vi "Main.vi"() -> ()   [LabVIEW 2013] (continued)
                n3208 = property on="Chart" class="WFChart (strict)"("History Data"=dynamicdata[] [[]]) -> (error out=w5362:errorcluster)  [unwired: 2 in, 1 out]
                n3209 = for {
                  N: w5364 -> [_]
                  i -> [w5373]
                  n3210 = property on="Chart" class="WFChart (strict)"("Active Plot"=w5373, "Plot.Plot Name"="") -> ()  [unwired: 2 in, 2 out]
                }
                n3211 = disable-structure shown="Disabled" {
                  disable-tunnel: w5362 -> [w5371 _]
                  frame Disabled {
                    # "1 hour"
                    n3212 = Get Date/Time In Seconds() -> (seconds since 1Jan1904=w5370:timestamp)
                    n3213 = To Double Precision Float(number=w5370) -> (double precision float=w5369:dbl)
                    n3214 = Add(x=w5369, y=3600.0) -> (x+y=w5367:dbl)
                    n3215 = property on="Chart" class="WFChart (strict)"(error in=w5371, "XScale.Minimum"=w5369, "XScale.Maximum"=w5367, "XScale.Increment"=1.0 ("X Scale.Range:Increment"), "XScale.ScaleFit"=u8 1 ("X Scale.Scale Fit")) -> ()  [unwired: 1 in, 2 out]
                  }
                  frame Enabled {
                  }
                }
              }
            }
            n3216 = property on="Recording Duration" class="DigNum (strict)"("Value"=0.0) -> ()  [unwired: 2 in, 2 out]
            n3217 = property on="Remaining Hold Time" class="DigNum (strict)"("Value"=w5354) -> ()  [unwired: 2 in, 2 out]
            n3218 = disable-structure shown="Disabled" {
              frame Disabled {
                # "Will be updated below"
                n3219 = local write "Raw Data File"("") -> ()
              }
              frame Enabled {
              }
            }
            n3220 = property on="Recipe Stop" class="Bool"("DisabledEnum"=T30."Enabled" ("Disabled")) -> ()  [unwired: 2 in, 2 out]
            n3221 = property on="Recipe Start" class="Bool"("DisabledEnum"=T30."Disabled and Grayed Out" ("Disabled")) -> ()  [unwired: 2 in, 2 out]
            n3222 = property on="Process Completed" class="Bool (strict)"("Colors [4]"=w5348, "Value"=FALSE ("Overall Status")) -> ()  [unwired: 2 in, 2 out]
            n3223 = property on="Hold Time Completed" class="Bool (strict)"("Colors [4]"=w5345, "Value"=FALSE ("Hold Time Completed")) -> ()  [unwired: 2 in, 2 out]
            n3224 = property on="Overall Status" class="Bool (strict)"("Colors [4]"=w5348, "Value"=FALSE ("Overall Status")) -> ()  [unwired: 2 in, 2 out]
          }
        }
        n3225 = local read "Probe List"() -> (w5224:i32[])
        n3226 = Path To String(path=w5209) -> (string=w5208:string)
        n3227 = Open/Create/Replace File(file path (use dialog)=w5209, error in=w5218, operation (0:open)=T41."replace or create") -> (refnum out=w5235:refnum<file>, error out=w5233:errorcluster)  [unwired: 3 in, 1 out]
        n3228 = Array To Spreadsheet String(delimiter (Tab)=",", array=w5224, 3:"%d" ("format string")) -> (spreadsheet string=w5220:string)
        n3229 = local write "Raw Data File"(w5208) -> ()
        n3230 = Concatenate Strings("Time," ("string"), w5220) -> (w5206:string)
        n3231 = case shown="True" "DB - Transaction" {
          tunnel: w5214 -> [_ w5297]
          tunnel: w5209 -> [_ w5291]
          tunnel: w5212 -> [_ w5288]
          tunnel: w5206 -> [_ w5252]
          frame False {
          }
          frame True {
            w5299 = T62[] [enum."[StartRecordTime]", enum."[PerformedBy]", enum."[PerformedOn]", enum."[RawDataFilePath]", enum."[RawDataFileName]", enum."[OutputSetId]", enum."[SavedBy]", enum."[SavedOn]"] items=["[StartRecordTime]", "[StartRecordTemp]", "[MaxRecordedTemp]", "[MaxRecordedTempTime]", "[MinRecordedTemp]", "[MinRecordedTempTime]", "[EndRecordTemp]", "[EndRecordTime]", "[RecordedMinutes]", "[StartHoldTime]", "[StartHoldTemp]", "[HoldTimeMaxTemp]", "[HoldTimeMaxTempTime]", "[HoldTimeMinTemp]", "[HoldTimeMinTempTime]", "[EndHoldTime]", "[EndHoldTemp]", "[HoldDurationMinutes]", "[TempDiffDuringHold]", "[UnitOfTemperature]", "[PerformedBy]", "[PerformedOn]", "[IsTempWithinTol]", "[IsTimeWithinTol]", "[HoldTimePercentage]", "[ProcessStatus]", "[OverallStatus]", "[SequenceStatus]", "[Parameter1]", "[Parameter2]", "[Parameter3]", "[Parameter4]", "[Parameter5]", "[Parameter6]", "[Parameter7]", "[Parameter8]", "[Parameter9]", "[Parameter10]", "[Parameter11]", "[Parameter12]", "[Result]", "[RawDataFile]", "[RawDataFilePath]", "[RawDataFileName]", "[OutputSetId]", "[SavedBy]", "[SavedOn]", "[Inactive]"] ("v02")
            # "<A> [PlantId]\n<B> [StationId]\n<C> [TransactionNo]\n<D> [TransactionRunNo]"
            # "Using SRTRS.Execute.Item instead of SRTRS.Setup.Item"
            # "EXEC GetNewTransactionRunNo to get the latest TransactionRunNo!!"
            # "INSERT [SRTRS].[Execute].[Header], [SRTRS].[Execute].[Item] [SRTRS].[Execute.][TransactionResult], [SRTRS].[Execute.][ProcedureItem], [SRTRS].[Execute.][Active], [CMS].[Execute.][ActiveProcess]"
            n3232 = local read "DB Refnums II"() -> (w5239:T24)
            n3233 = local read "DB Refnums"() -> (w5278:T23)
            n3234 = call "DB - [Execute].[Transaction].vi"("DB.Schema.Table"="SRTRS.Execute.Header", "Transaction"=w5297, "error in (no error)"=errorcluster {"status"=FALSE, "code"=0, "source"=""}, "DB Connection"=T53 {"Open"=TRUE, "Close"=FALSE}, "Refnums"=w5278, "DB - Execute Transaction"=DB_-_Execute_Transaction_Enum."INSERT INTO [Header]" ("DB - Setup Item Enum"), "DB Refnums II"=w5239) -> ("connection reference"=w5251:T66, "Transaction"=w5284:T19, "SUMMARY"=w5283:errorcluster)  [unwired: 9 in, 1 out]
            n3235 = Unbundle By Name(w5284) -> ("TransactionRunNo"=w5273:string)
            n3236 = local write "TransactionRunNo"(w5273) -> ()
            n3237 = local write "TransactionRunNo (Execute)"(w5273) -> ()
            n3238 = global write "Global SRTRS.vi" "[TransactionRunNo]"(w5273) -> ()
            n3239 = Build Array("SRTRS.Execute.Item" ("DB.Schema.Table")) -> (w5276:string[])
            n3240 = call "DB - [Setup].[Item] (Part Details).vi"("DB - Setup Item Enum"=DB_-_Setup_Item_Enum."INSERT [Setup].[Item]", "DB.Schema.Table Array"=w5276, "Transaction"=w5284, "error in (no error)"=w5283, "DB Refnums"=w5278) -> ("Transaction"=w5281:T19, "SUMMARY"=w5282:errorcluster)  [unwired: 5 in, 4 out]
            n3241 = Strip Path(path=w5291) -> (stripped path=w5290:path, name=w5287:string)
            n3242 = Path To String(path=w5290) -> (string=w5264:string)
            n3243 = call "DB - [Execute].[Transaction].vi"("connection reference"=w5251, "DB.Schema.Table"="SRTRS.Execute.TransactionResult", "Transaction"=w5281, "error in (no error)"=w5282, "DB Connection"=T53 {"Open"=FALSE, "Close"=FALSE}, "Refnums"=w5278, "DB - Execute Transaction"=DB_-_Execute_Transaction_Enum."INSERT INTO [TransactionResult]" ("DB - Setup Item Enum"), "DB Refnums II"=w5239) -> ("connection reference"=w5250:T66, "Transaction"=w5286:T19, "SUMMARY"=w5293:errorcluster)  [unwired: 8 in, 1 out]
            n3244 = Concatenate Strings(w5264, "\\" ("string")) -> (w5262:string)
            n3245 = call "DB - [Execute].[Transaction].vi"("connection reference"=w5250, "DB.Schema.Table"="SRTRS.Execute.ProcedureItem", "Transaction"=w5286, "error in (no error)"=w5293, "DB Connection"=T53 {"Open"=FALSE, "Close"=FALSE}, "Refnums"=w5278, "DB - Execute Transaction"=DB_-_Execute_Transaction_Enum."INSERT INTO [ProcedureItem]" ("DB - Setup Item Enum"), "DB Refnums II"=w5239) -> ("connection reference"=w5249:T66, "Transaction"=w5285:T19, "SUMMARY"=w5292:errorcluster)  [unwired: 8 in, 1 out]
            n3246 = global read "Global SRTRS.vi" "Date Time Format"() -> (w5289:string)
            n3247 = global read "Global SRTRS.vi" "Logon"() -> (w5269:T21)
            n3248 = Unbundle By Name(w5269) -> ("UserID"=w5275:string)
            n3249 = Format Date/Time String(time format string (%c)=w5289, seconds (now)=w5288) -> (date/time string=w5256:string)  [unwired: 1 in]
            "[StartRecordTime]" <- w5256
            n3250 = property on="Output Set" class="CmbBox (strict)"() -> ("Value"=w5242:T5)  [unwired: 2 in, 2 out]
            n3251 = Build Array(w5256, w5275, w5256, w5262, w5287, w5242, w5275, w5256) -> (w5298:T5[])
            n3252 = call "DB - [Execute].[Transaction].vi"("connection reference"=w5249, "DB.Schema.Table"="SRTRS.Execute.TransactionResult", "Transaction"=w5285, "error in (no error)"=w5292, "DB Connection"=T53 {"Open"=FALSE, "Close"=FALSE}, "DB - Execute Transaction"=DB_-_Execute_Transaction_Enum."UPDATE [TransactionResult]" ("DB - Setup Item Enum"), "[TransactionResult] v02"=w5299, "<Values>"=w5298) -> ("connection reference"=w5248:T66, "Transaction"=w5266:T19, "SUMMARY"=w5272:errorcluster)  [unwired: 8 in, 1 out]
            n3253 = Unbundle By Name(w5266) -> ("TransactionNo"=w5258:string, "TransactionRunNo"=w5257:string)
            n3254 = Unbundle By Name(w5269) -> ("PlantID"=w5268:string, "StationID"=w5267:string)
            n3255 = local read "Enable Central Monitoring"() -> (w5261:bool)
            n3256 = Build Array(w5268, w5267, w5258, w5257) -> (w5265:string[])
            n3257 = call "DB - [Execute].[Transaction].vi"("connection reference"=w5248, "DB.Schema.Table"="SRTRS.Execute.Active", "error in (no error)"=w5272, "DB Connection"=T53 {"Open"=FALSE, "Close"=TRUE}, "DB - Execute Transaction"=DB_-_Execute_Transaction_Enum."INSERT/UPDATE [Execute].[Active]", "<Values>"=w5265) -> ("SUMMARY"=w5253:errorcluster)  [unwired: 10 in, 3 out]
            n3258 = And(x=w5261, y="DB - Active Process") -> (x .and. y?=w5260:bool)
            n3259 = case shown="True" w5260 {
              tunnel: [_ w5318] -> w5255
              tunnel: w5258 -> [_ w5331]
              tunnel: w5257 -> [_ w5330]
              tunnel: w5256 -> [_ w5310]
              tunnel: w5253 -> [_ _]
              tunnel: w5252 -> [_ w5315]
              frame False {
              }
              frame True {
                w5316 = "0"  # Start at Beginning
                w5332 = T63[] [enum."[IsActive]", enum."[TransactionNo]", enum."[TransactionRunNo]", enum."[StartRecordTime]", enum."[HoldProgressColor]", enum."[ProcessColor]", enum."[OverallColor]"] items=["[IsActive]", "[TransactionNo]", "[TransactionRunNo]", "[SequenceStatus]", "[StartRecordTime]", "[EndRecordTime]", "[StartHoldTime]", "[EndHoldTime]", "[Message1]", "[Message2]", "[HoldTimeRemaining]", "[HoldTimePercentage]", "[HoldProgressColor]", "[OrderNumbers]", "[CurrentTemp]", "[UnitOfTemperature]", "[IsAppClientLive]", "[RawDataFile]", "[RecordedMinutes]", "[FurnaceControlStatus]", "[FurnaceControlColor]", "[ControllerStatus]", "[ControllerColor]", "[IsControllerOnline]", "[ProcessColor]", "[OverallColor]", "[LastUpdatedOn]", "[LastUpdatedCmsTime]", "[Inactive]"] ("[Execute].[ActiveProcess]\n2014-10-14 14:58")
                n3260 = global read "Global SRTRS.vi" "Logon"() -> (w5336:T21)
                n3261 = Unbundle By Name(w5336) -> ("PlantID"=w5328:string, "SystemID"=w5327:string)
                n3262 = control-ref of="Hold Time Completed"() -> (w5309:refnum<vi>)
                n3263 = control-ref of="Overall Status"() -> (w5312:refnum<vi>)
                n3264 = control-ref of="Process Completed"() -> (w5313:refnum<vi>)
                n3265 = Bundle("PlantID"=w5328, "SystemID"=w5327) -> (w5317:cluster{"PlantID":string, "SystemID":string})  [unwired: 1 in]
                n3266 = call "DB - [CMS].[Execute].[ActiveProcess].vi"("Application"="SRTRS", "[PlantId],[SystemId]"=w5317, "DB Connection"=T53 {"Open"=TRUE, "Close"=FALSE}, "DB - CMS Execute ActiveProcess"=DB_-_CMS_Execute_Active_Process."INSERT INTO [Execute].[ActiveProcess]") -> ("connection reference"=w5326:T66, "SUMMARY"=w5335:errorcluster)  [unwired: 12 in, 2 out]
                n3267 = call "String - Boolean Ref Color.vi"("Bool Refnum"=w5313) -> ("Color (U32 String)"=w5314:string)  [unwired: 4 in]
                n3268 = call "String - Boolean Ref Color.vi"("Bool Refnum"=w5312) -> ("Color (U32 String)"=w5311:string)  [unwired: 4 in]
                n3269 = call "String - Boolean Ref Color.vi"("Bool Refnum"=w5309) -> ("Color (U32 String)"=w5308:string)  [unwired: 4 in]
                n3270 = Build Array("1" ("element"), w5331, w5330, w5310, w5308, w5314, w5311) -> (w5329:string[])
                n3271 = call "DB - [CMS].[Execute].[ActiveProcess].vi"("connection reference"=w5326, "Application"="SRTRS", "[PlantId],[SystemId]"=w5317, "error in (no error)"=w5335, "DB Connection"=T53 {"Open"=FALSE, "Close"=FALSE}, "DB - CMS Execute ActiveProcess"=DB_-_CMS_Execute_Active_Process."UPDATE [Execute].[ActiveProcess]", "[Execute].[ActiveProcess]\n2014-10-14 14:58"=w5332, "<Data>"=w5329) -> ("connection reference"=w5320:T66, "SUMMARY"=w5319:errorcluster)  [unwired: 8 in, 2 out]
                n3272 = call "DB - [CMS].[Execute].[ActiveProcess].vi"("connection reference"=w5320, "Application"="SRTRS", "String ([RawDataFile] Filestream)"=w5315, "[PlantId],[SystemId]"=w5317, "error in (no error)"=w5319, "DB Connection"=T53 {"Open"=FALSE, "Close"=TRUE}, "Filestream Position (0/<int>/NULL)"=w5316, "DB - CMS Execute ActiveProcess"=DB_-_CMS_Execute_Active_Process."UPDATE FILESTREAM") -> ("SUMMARY"=w5318:errorcluster)  [unwired: 8 in, 3 out]
              }
            }
            n3273 = Merge Errors(w5255, w5253) -> (w5254:errorcluster)
            n3274 = case shown="Error" w5254 {
              tunnel: " /* [SRTRS].[Execute].[Item,TransactionResult,ProcedureItem,TransactionResult], [CMS].[Execute].[ActiveProcess]*/" ("Message") -> [w5338 w5341]
              tunnel: [w5337 w5340] -> w5241
              frame No Error {
                n3275 = Concatenate Strings("{Start Recipe} Transaction DB Record Create OK." ("string"), w5338) -> (w5337:string)
              }
              frame Error {
                n3276 = Concatenate Strings("{Start Recipe} Transaction DB Record Create Failed." ("string"), w5341) -> (w5340:string)
              }
            }
            n3277 = call "Queue - EnQueue to MessageQ.vi"("<NoD> Don't Display to UI"=TRUE, "Message"=w5241) -> ()  [unwired: 9 in, 1 out]
            n3278 = local write "DB"(w5254) -> ()
          }
        }
        n3279 = Write to Text File(file (use dialog)=w5235, text=w5206, error in=w5233) -> (refnum out=→"Logged File Ref":refnum<file>, error out=w5228:errorcluster)  [unwired: 1 in, 1 out]
        "Data File Error" <- w5228
        n3280 = case shown="No Error" w5228 {
          tunnel: w5207 -> [w5386 _]
          tunnel: [w5382 "{Start Recipe} Raw Data File Create Failed." ("string")] -> w5205
          frame No Error {
            w5385 = "\""
            # "Display on Front Panel"
            n3281 = local write "Raw Data File"(w5386) -> ()
            n3282 = Concatenate Strings(w5385, w5386, w5385) -> (w5378:string)
            n3283 = call <vilib>:"Application Directory.vi"() -> ("Application Directory"=w5390:path)
            n3284 = Build Path(base path=w5390, name or relative path="SRTRS.ini" ("ini Name")) -> (appended path=w5391:path)
            n3285 = call <vilib>:"Open Config Data.vi"("create file if necessary (T)"=FALSE, "configuration file path"=w5391) -> ("error out"=w5388:errorcluster, "refnum"=w5389:T59)  [unwired: 7 in, 1 out]
            n3286 = call-poly <vilib>:"Write Key.vi"("write raw string? (F)"=TRUE, "section"="Settings", "error in (no error)"=w5388, "value"=w5386, "key"="Raw Data File", "refnum"=w5389) -> ("error out"=w5394:errorcluster, "found?"=w5395:bool, "refnum out"=w5396:T59)  [unwired: 3 in]
            n3287 = call "Msgbox - Message Handler.vi"("Short Description (When DB Not Available)"="Process Started", "Description (When DB Not Available)"="Process started successfully. Raw data is logging to " ("Short Description (When DB Not Available)"), "Post-Description"=w5378, "<.?....> Message Code"="<I 303>") -> ("MHandler Error"=w5377:errorcluster)  [unwired: 5 in, 2 out]
            n3288 = local write "MHandler"(w5377) -> ()
            n3289 = call <vilib>:"Close Config Data.vi"("error in (no error)"=w5394, "write file if changed (T)"=w5395, "refnum"=w5396) -> ("error out"=w5384:errorcluster)  [unwired: 7 in, 1 out]
            n3290 = local write "ini File Error"(w5384) -> ()
            n3291 = Concatenate Strings("{Start Recipe} Raw Data File Created: " ("string"), w5378) -> (w5382:string)
          }
          frame Error {
          }
        }
        n3292 = call "Queue - EnQueue to MessageQ.vi"("<NoD> Don't Display to UI"=TRUE, "Message"=w5205) -> ()  [unwired: 9 in, 1 out]
      }
      frame "START Recovery" {
        w5426 = T62[] [enum."[RawDataFilePath]", enum."[RawDataFileName]", enum."[StartHoldTime]", enum."[EndHoldTime]", enum."[HoldTimePercentage]", enum."[StartHoldTemp]", enum."[EndHoldTemp]"] items=["[StartRecordTime]", "[StartRecordTemp]", "[MaxRecordedTemp]", "[MaxRecordedTempTime]", "[MinRecordedTemp]", "[MinRecordedTempTime]", "[EndRecordTemp]", "[EndRecordTime]", "[RecordedMinutes]", "[StartHoldTime]", "[StartHoldTemp]", "[HoldTimeMaxTemp]", "[HoldTimeMaxTempTime]", "[HoldTimeMinTemp]", "[HoldTimeMinTempTime]", "[EndHoldTime]", "[EndHoldTemp]", "[HoldDurationMinutes]", "[TempDiffDuringHold]", "[UnitOfTemperature]", "[PerformedBy]", "[PerformedOn]", "[IsTempWithinTol]", "[IsTimeWithinTol]", "[HoldTimePercentage]", "[ProcessStatus]", "[OverallStatus]", "[SequenceStatus]", "[Parameter1]", "[Parameter2]", "[Parameter3]", "[Parameter4]", "[Parameter5]", "[Parameter6]", "[Parameter7]", "[Parameter8]", "[Parameter9]", "[Parameter10]", "[Parameter11]", "[Parameter12]", "[Result]", "[RawDataFile]", "[RawDataFilePath]", "[RawDataFileName]", "[OutputSetId]", "[SavedBy]", "[SavedOn]", "[Inactive]"] ("[TransactionResult] v02")
        w5427 = T35 [enum."Page Disabled & Grayed", enum."Page Enabled", enum."Page Disabled & Grayed", enum."Page Disabled & Grayed", enum."Page Enabled"] items=["Page Enabled", "Page Disabled", "Page Disabled & Grayed"]
        # "Recovery"
        n3293 = property on="Tab Body" class="TabCtl (strict)"() -> ("Pages"=w5428:refnum<vi>[])  [unwired: 2 in, 2 out]
        n3294 = for {
          tunnel: w5428 -> [w5564] mode=indexing
          tunnel: w5427 -> [w5563] mode=indexing
          n3295 = property class="Page"(reference=w5564, "PageEnb"=w5563) -> ()  [unwired: 1 in, 2 out]
        }
        n3296 = local read "Data Path Name (cRIO SV)"() -> (w5414:string)
        n3297 = local read "Simulate cRIO"() -> (w5416:bool)
        n3298 = local read "Data_Host"() -> (w5417:path)
        n3299 = global read "Global SRTRS.vi" "[TransactionRunNo]"() -> (w5419:string)
        n3300 = global read "Global SRTRS.vi" "[TransactionNo]"() -> (w5420:string)
        n3301 = Bundle("[TransactionNo]"=w5420, "[TransactionRunNo]"=w5419) -> (w5421:T60)  [unwired: 1 in]
        n3302 = call "DB - [Execute].[Transaction].vi"("DB.Schema.Table"="SRTRS.Execute.TransactionResult", "Transaction"=w5421, "DB - Execute Transaction"=DB_-_Execute_Transaction_Enum."SELECT [TransactionResult]", "[TransactionResult] v02"=w5426) -> ("1D Results"=w5424:string[], "SUMMARY"=w5405:errorcluster)  [unwired: 12 in, 2 out]
        n3303 = local write "DB"(w5405) -> ()
        n3304 = Index Array(array=w5424) -> (element #1=w5423:string, element #2=w5422:string, element #3=w5409:string, element #4=w5408:string, element #5=w5412:string, element #6=w5407:string, element #7=w5406:string)  [unwired: 7 in]
        n3305 = Concatenate Strings(w5423, w5422) -> (w5413:string)
        n3306 = local write "Raw Data File"(w5413) -> ()
        n3307 = case shown="True" w5416 {
          tunnel: w5413 -> [w5485 w5519]
          tunnel: [w5500 w5527] -> w5415
          tunnel: [w5497 errorcluster {"status"=FALSE, "code"=0, "source"="FTP Skipped"} ("error out")] -> w5400
          tunnel: w5417 -> [w5498 _]
          tunnel: w5414 -> [w5494 _]
          frame False {
            w5479 = "\"" ("string")
            w5483 = "\"" ("string")
            # "Should Match with Raw Data File Stored in ini\nMatching ONLY the name"
            # "Change \n/c/ni-rt/LabVIEW Data/SRTRS4070/Data/2014/08/0090300742_20140822_114859.dat\nTO\nc:\\ni-rt\\LabVIEW Data\\SRTRS4070\\Data\\2014\\04\\0090300742_20140822_114859.dat"
            # "FTP Raw Data File  from cRIO AND \nReplaces data file in Data_Host\nSimilar Step as {END Recipe}"
            n3308 = Search and Replace String(replace all?=TRUE ("replace all? (F)"), input string=w5494, search string="/", replace string="\\" ("replace string (\"\")")) -> (result string=w5503:string)  [unwired: 4 in, 3 out]
            n3309 = String To Path(string=w5485) -> (path=w5487:path)
            n3310 = Strip Path "<>.dat"(path=w5487) -> (name=w5486:string)  [unwired: 1 out]
            n3311 = Search and Replace String(input string=w5503, search string="\\c", replace string="c:" ("replace string (\"\")")) -> (result string=w5478:string)  [unwired: 5 in, 3 out]
            n3312 = String To Path(string=w5478) -> (path=w5499:path)
            n3313 = Strip Path "<>.dat"(path=w5499) -> (name=w5493:string)  [unwired: 1 out]
            n3314 = Equal?(x=w5493, y=w5486) -> (x = y?=w5492:bool)
            "SV and ini Data File Name Match. (Recovery)" <- w5492
            n3315 = Build Path(base path=w5498, name or relative path=w5493) -> (appended path=w5500:path)
            n3316 = Concatenate Strings(w5479, w5478, w5479) -> (w5477:string)
            n3317 = local read "cRIO IP"() -> (w5507:string)
            n3318 = call <vilib>:"FTP Get File.vi"("password"="", "user"="anonymous", "local path"=w5500, "remote path"=w5478, "host"=w5507) -> ("error out"=w5497:errorcluster)  [unwired: 5 in, 1 out]
            n3319 = case shown="No Error" w5497 {
              tunnel: ["{Start Recovery} FTP OK. " "{Start Recovery} FTP failed. "] -> w5495
              tunnel: ["<I 321>" ("<.?....> Message Code") "<E 322>" ("<.?....> Message Code")] -> w5480
              tunnel: ["Raw Data Loaded Successfully" ("<.?....> Message Code") "Raw Data Load Failed" ("<.?....> Message Code")] -> w5476
              tunnel: [" is loaded." ("<.?....> Message Code") " cannot be loaded." ("<.?....> Message Code")] -> w5475
              frame No Error {
              }
              frame Error {
              }
            }
            n3320 = Select(t=". SV and ini Data File Name Match. ", s=w5492, f=". SV and ini Data File Name does not Match. ") -> (s? t:f=w5488:string)
            n3321 = call "Msgbox - Message Handler.vi"("Short Description (When DB Not Available)"=w5476, "Description (When DB Not Available)"=w5475, "Pre-Description"=w5477, "<.?....> Message Code"=w5480) -> ("MHandler Error"=w5481:errorcluster)  [unwired: 5 in, 2 out]
            n3322 = Concatenate Strings(w5495, "cRIO File: " ("string"), w5477, " ini File: " ("string"), w5483, w5485, w5483, w5488) -> (w5482:string)
            n3323 = local write "MHandler"(w5481) -> ()
            n3324 = call "Queue - EnQueue to MessageQ.vi"("<NoD> Don't Display to UI"=TRUE, "Message"=w5482) -> ()  [unwired: 9 in, 1 out]
          }
          frame True {
            w5521 = "\"" ("string")
            # "c:\\temp\\SRTRS4070_Host\\Data_Host\\2014\\08\\0090300742_20140822_114859.dat"
            # "Skip FTP in Simulate cRIO Mode\nRaw Data file is using the original data file in Data_Host"
            n3325 = String To Path(string=w5519) -> (path=w5527:path)
            n3326 = Concatenate Strings(w5521, w5519, w5521, " (Simulated)" ("string")) -> (w5520:string)
            n3327 = call "Msgbox - Message Handler.vi"("Short Description (When DB Not Available)"="Raw Data Loaded Successfully" ("<.?....> Message Code"), "Description (When DB Not Available)"=" is loaded." ("<.?....> Message Code"), "Pre-Description"=w5520, "<.?....> Message Code"="<I 321>") -> ("MHandler Error"=w5525:errorcluster)  [unwired: 5 in, 2 out]
            n3328 = call "Queue - EnQueue to MessageQ.vi"("<NoD> Don't Display to UI"=TRUE, "Message"="{Start Recovery} FTP skipped in cRIO Simulate Mode. ") -> ()  [unwired: 9 in, 1 out]
            n3329 = local write "MHandler"(w5525) -> ()
          }
        }
        n3330 = local read "DB - Active Process"() -> (w5403:bool)
        n3331 = local read "Enable Central Monitoring"() -> (w5404:bool)
        n3332 = flat-sequence "EXECUTE TAB" {
          tunnel: w5409 -> [w5542]
          tunnel: w5408 -> [w5541]
          tunnel: w5412 -> [w5538]
          frame #0 {
            w5544 = T36 [{"Color Box"=9868950, "Color Box 2"=9868950}, {"Color Box"=6618880, "Color Box 2"=6618880}, {"Color Box"=4934475, "Color Box 2"=4934475}, {"Color Box"=6618880, "Color Box 2"=6618880}]  # Init
            w5545 = T36 [{"Color Box"=9868950, "Color Box 2"=9868950}, {"Color Box"=6618880, "Color Box 2"=6618880}, {"Color Box"=4934475, "Color Box 2"=4934475}, {"Color Box"=6618880, "Color Box 2"=6618880}]  # Init
            w5547 = cluster{"Color Box":u32, "Color Box 2":u32}[] [{"Color Box"=16383786, "Color Box 2"=16383786}, {"Color Box"=6618880, "Color Box 2"=6618880}, {"Color Box"=4934475, "Color Box 2"=4934475}, {"Color Box"=6618880, "Color Box 2"=6618880}]  # Start Recipe
            # "Jump to Execute TAB\nThis is used when SRTRS is\nrecovered"
            # "\"START Recovery\""
            n3333 = Fract/Exp String To Number(string=w5538) -> (number=w5530:dbl)  [unwired: 3 in, 1 out]
            n3334 = call "String - Convert Str (YYYY-mm-dd HHcMMcSS) to TimeStamp.vi"("YYYY-mm-dd HH:MM:SS (String)"=w5542) -> ("time stamp"=w5540:timestamp)  [unwired: 9 in, 1 out]
            n3335 = call "String - Convert Str (YYYY-mm-dd HHcMMcSS) to TimeStamp.vi"("YYYY-mm-dd HH:MM:SS (String)"=w5541) -> ("time stamp"=w5539:timestamp)  [unwired: 9 in, 1 out]
            n3336 = Greater Or Equal?(x=w5530, y=99.5) -> (x >= y?=w5536:bool)
            n3337 = Greater?(x=w5530, y=0.0) -> (0:w5534:bool)
            n3338 = property on="Variant Allowed (Hold Temp)" class="Bool (strict)"("Colors [4]"=w5545, "Value"=FALSE) -> ()  [unwired: 2 in, 2 out]
            n3339 = local write "% Hold. Time Completed (Num)"(w5530) -> ()
            n3340 = local write "Parameter (Start Dwell Time)"(w5540) -> ()
            n3341 = local write "Parameter (End Dwell Time)"(w5539) -> ()
            n3342 = property on="Variant Allowed (Hold Time)" class="Bool (strict)"("Colors [4]"=w5545, "Value"=FALSE) -> ()  [unwired: 2 in, 2 out]
            n3343 = Select(t=u32 786176 ("Fill Color"), s=w5534, f=u32 16777216 ("Color Box 2")) -> (s? t:f=w5531:u32)
            n3344 = property on="% Hold. Time Completed" class="Slide (strict)"("Scale.Maximum"=100.0 ("Scale.Range:Maximum"), "Scale.Minimum"=0.0 ("Scale.Range:Minimum"), "Fill Color"=w5531, "Value"=w5530) -> ()  [unwired: 2 in, 2 out]
            n3345 = property on="Hold. Time (hour:minute)" class="Str"() -> ("Value"=w5555:string)  [unwired: 2 in, 2 out]
            n3346 = property on="Tab Body" class="TabCtl (strict)"("Value"=Enum_-_Tabs."Execute" ("Tab Body")) -> ()  [unwired: 2 in, 2 out]
            n3347 = call "String - Format to (HH_colon_MM).vi"("xx:xx"=w5555) -> ("seconds"=w5553:dbl)  [unwired: 9 in, 1 out]
            n3348 = flat-sequence {
              frame #0 {
                w5559 = 12  # 12 Probes Max
                n3349 = property on="Chart" class="WFChart (strict)"("History Data"=dynamicdata[] []) -> ()  [unwired: 2 in, 2 out]
                n3350 = for {
                  N: w5559 -> [_]
                  i -> [w5561]
                  n3351 = property on="Chart" class="WFChart (strict)"("Active Plot"=w5561, "Plot.Plot Name"="") -> ()  [unwired: 2 in, 2 out]
                }
              }
            }
            n3352 = property on="Recording Duration" class="DigNum (strict)"("Value"=0.0) -> ()  [unwired: 2 in, 2 out]
            n3353 = property on="Remaining Hold Time" class="DigNum (strict)"("Value"=w5553) -> ()  [unwired: 2 in, 2 out]
            n3354 = disable-structure shown="Disabled" {
              frame Disabled {
                # "Will be updated below"
                n3355 = local write "Raw Data File"("") -> ()
              }
              frame Enabled {
              }
            }
            n3356 = property on="Recipe Stop" class="Bool"("DisabledEnum"=T30."Enabled" ("Disabled")) -> ()  [unwired: 2 in, 2 out]
            n3357 = property on="Recipe Start" class="Bool"("DisabledEnum"=T30."Disabled and Grayed Out" ("Disabled")) -> ()  [unwired: 2 in, 2 out]
            n3358 = property on="Hold Time Completed" class="Bool (strict)"("Colors [4]"=w5544, "Value"=w5536) -> ()  [unwired: 2 in, 2 out]
            n3359 = property on="Process Completed" class="Bool (strict)"("Colors [4]"=w5547, "Value"=FALSE ("Overall Status")) -> ()  [unwired: 2 in, 2 out]
            n3360 = property on="Overall Status" class="Bool (strict)"("Colors [4]"=w5547, "Value"=FALSE ("Overall Status")) -> ()  [unwired: 2 in, 2 out]
          }
        }
        n3361 = Bundle By Name(cluster=T15 {"Start Holding Time and Date"="", "End Holding Time and Date"="", "Start Holding Temperature"="", "End Holding Temperature"=""} ("Parameter Buffer"), "Start Holding Time and Date"=w5409, "End Holding Time and Date"=w5408, "Start Holding Temperature"=w5407, "End Holding Temperature"=w5406) -> (w5410:T15)
        n3362 = And(x=w5404, y=w5403) -> (x .and. y?=w5402:bool)
        n3363 = property on="Parameter Buffer" class="Clust (strict)"("Value"=w5410) -> ()  [unwired: 2 in, 2 out]
        n3364 = case shown="No Error" w5400 {
          selector: w5400 -> [_ w5474]
          tunnel: w5415 -> [w5462 _]
          tunnel: [w5459 w5474] -> _
          tunnel: [w5454 refnum<file> refnum ("refnum")] -> w5401
          frame No Error {
            w5460 = "\n"
            w5449 = "\"" ("string")
            # "Shift Pointer to End of File"
            # "Overwrite raw data from cRIO to Chart"
            n3365 = call "Chart - Load History.vi"("file path (dialog if empty)"=w5462) -> ("Error Out"=w5465:errorcluster, "History"=w5466:dynamicdata[], "size(s)"=→"Recovered Data Size":i32[])  [unwired: 5 in, 3 out]
            n3366 = Path To String(path=w5462) -> (string=w5450:string)
            n3367 = property on="Chart" class="WFChart (strict)"(error in=w5465, "History Data"=w5466) -> (error out=w5459:errorcluster)  [unwired: 1 in, 1 out]
            n3368 = Open/Create/Replace File(file path (use dialog)=w5462, error in=w5459, operation (0:open)=T41."open or create") -> (refnum out=w5456:refnum<file>, error out=w5458:errorcluster)  [unwired: 3 in, 1 out]
            n3369 = Set File Position(refnum=w5456, from (0:start)=enum16{"start", "end", "current"}."end", error in=w5458) -> (refnum out=w5454:refnum<file>, error out=w5457:errorcluster)  [unwired: 1 in]
            n3370 = local write "Logged File Ref"(w5454) -> ()
            n3371 = case shown="No Error" w5459 {
              tunnel: ["Raw Data File Load to Chart OK. " "Raw Data File Load to Chart failed. "] -> w5464
              frame No Error {
              }
              frame Error {
              }
            }
            n3372 = case shown="No Error" w5457 {
              tunnel: ["Open for Logging OK." "Open for Logging Failed."] -> w5461
              frame No Error {
              }
              frame Error {
              }
            }
            n3373 = Merge Errors(w5457, w5459) -> (w5452:errorcluster)
            n3374 = local write "Data File Error"(w5452) -> ()
            n3375 = case shown="No Error" w5452 {
              tunnel: ["<I 321>" ("<.?....> Message Code") "<E 322>" ("<.?....> Message Code")] -> _
              frame No Error {
              }
              frame Error {
              }
            }
            n3376 = Concatenate Strings(w5449, w5450, w5449) -> (w5446:string)
            n3377 = Concatenate Strings("{Start Recovery}" ("string"), w5461, w5460, w5464, w5460, w5446) -> (w5447:string)
            n3378 = call "Queue - EnQueue to MessageQ.vi"("<NoD> Don't Display to UI"=TRUE, "Message"=w5447) -> ()  [unwired: 9 in, 1 out]
          }
          frame Error {
          }
        }
        n3379 = case shown="True" w5402 {
          tunnel: w5401 -> [_ w5435]
          tunnel: w5400 -> [_ w5432]
          frame False {
          }
          frame True {
            # "Load cRIO's Data File to [Execute].[ActiveProcess]"
            n3380 = Set File Position(refnum=w5435, from (0:start)=enum16{"start", "end", "current"}."start", error in=w5432) -> (refnum out=w5444:refnum<file>, error out=w5443:errorcluster)  [unwired: 1 in]
            n3381 = Read from Text File(file (use dialog)=w5444, count=-1, error in=w5443) -> (text=w5434:string, error out=w5431:errorcluster)  [unwired: 1 in, 2 out]
            n3382 = local write "Data File Error"(w5431) -> ()
            n3383 = global read "Global SRTRS.vi" "Logon"() -> (w5438:T21)
            n3384 = Unbundle By Name(w5438) -> ("PlantID"=w5439:string, "SystemID"=w5440:string)
            n3385 = Bundle("PlantID"=w5439, "SystemID"=w5440) -> (w5441:cluster{"PlantID":string, "SystemID":string})  [unwired: 1 in]
            n3386 = call "DB - [CMS].[Execute].[ActiveProcess].vi"("Application"="SRTRS", "String ([RawDataFile] Filestream)"=w5434, "[PlantId],[SystemId]"=w5441, "error in (no error)"=w5431, "Filestream Position (0/<int>/NULL)"="0", "DB - CMS Execute ActiveProcess"=DB_-_CMS_Execute_Active_Process."UPDATE FILESTREAM") -> ("SUMMARY"=w5433:errorcluster)  [unwired: 10 in, 3 out]
            n3387 = local write "DB"(w5433) -> ()
          }
        }
      }
      frame "BEGIN Process" {
        # "Intialize ET3500"
        # "START DAQ, START MONITORING ET3504\nUPDATE Sequence Status\nSET Process t0 (used for relative time stamp in Raw Data File)\nReset RecoveryFlag?"
        n3388 = local read "cRIO DAQ Started"() -> (w5568:bool)
        n3389 = case shown="False" w5568 {
          tunnel: [w5609 _] -> w5577
          frame False {
            w5614 = TRUE  # DAQ Start
            # "Create Transaction No"
            # "Start DAQ"
            # "Not Started Yet"
            n3390 = local read "cRIO Folder"() -> (w5603:string)
            n3391 = Format Date/Time String(time format string (%c)="/%Y/%m/") -> (date/time string=w5606:string)  [unwired: 2 in]
            n3392 = Concatenate Strings(w5603, "/Data" ("string"), w5606) -> (w5607:string)
            n3393 = disable-structure shown="Enabled" {
              disable-tunnel: w5607 -> [w5621 w5623]
              disable-tunnel: [w5615 w5626] -> w5602
              frame Disabled {
                # "May have 1-2 seconds of difference, since the host\nfile time was created in the previous state"
                n3394 = local read "Transaction No"() -> (w5616:string)
                n3395 = Format Date/Time String(time format string (%c)="%Y%m%d_%H%M%S") -> (date/time string=w5618:string)  [unwired: 2 in]
                n3396 = Concatenate Strings(w5621, w5616, "_" ("string"), w5618, ".dat" ("string")) -> (w5615:string)
              }
              frame Enabled {
                n3397 = local read "Raw Data File"() -> (w5624:string)
                n3398 = String To Path(string=w5624) -> (path=w5625:path)
                n3399 = Strip Path(path=w5625) -> (name=w5622:string)  [unwired: 1 out]
                n3400 = Concatenate Strings(w5623, w5622) -> (w5626:string)
              }
            }
            n3401 = local read "cRIO Channel List"() -> (w5601:i32[])
            n3402 = local read "Simulate cRIO"() -> (w5610:bool)
            n3403 = local read "cRIO shared variable RT Library"() -> (w5612:string)
            n3404 = local read "Probe List"() -> (w5611:i32[])
            n3405 = control-ref of="cRIO Status"() -> (w5608:refnum<vi>)
            n3406 = call "cRIO - Shared Variable RW.vi"("shared variable RT Library"=w5612, "Read/Write"=cRIO_RW_Enum."Write", "Data Path Name"=w5602, "cRIO Channel List (In)"=w5601, "Simulate cRIO"=w5610, "Probe List In"=w5611, "DAQ Start"=w5614, "cRIO Status"=w5608) -> ("Error Out"=w5609:errorcluster)  [unwired: 3 in, 8 out]
          }
          frame True {
            # "Already Started in \"Ready to Start\" \ni.e. PC crashed in previous run\nSo no need to resend DAQ Start"
          }
        }
        n3407 = flat-sequence {
          tunnel: w5583 -> [w5600]
          tunnel: w5577 -> [_]
          frame #0 {
            # "Shows on UI:\n\"Applicatoin Logging Started\"  /* The rest are commented out  */"
            # "EnQ MessageQ"
            n3408 = Number To Fractional String(number=w5600, precision (6)=i16 1) -> (F-format string=w5597:string)  [unwired: 2 in]
            n3409 = local read "ET3504 Status"() -> (w5594:string)
            n3410 = local read "cRIO Status"() -> (w5593:string)
            n3411 = Concatenate Strings("{BEGIN Process} ", "PVin = ", w5597, ". ET Status: " ("string"), w5594, ". cRIO Status: " ("string"), w5593) -> (w5591:string)
            n3412 = call "Queue - EnQueue to MessageQ.vi"("<NoD> Don't Display to UI"=TRUE, "Message"=w5591) -> ()  [unwired: 9 in, 1 out]
          }
        }
        n3413 = local read "VISA resource name RS232"() -> (w5587:string)
        n3414 = local read "Simulate ET3500"() -> (w5585:bool)
        n3415 = control-ref of="ET3504 Status"() -> (w5567:refnum<vi>)
        n3416 = local write "cRIO Error"(w5577) -> ()
        n3417 = call "ET3500 - Read Program Parameters.vi"("Simulate"=w5585, "ET3500 Status"=w5567, "subVI (Auto Interactive)"=TRUE ("subVI"), "Option"=cluster{"Init":bool, "Close":bool} {"Init"=TRUE, "Close"=FALSE}, "VISA resource name"=w5587) -> ("error out"=w5579:errorcluster, "Segment.Type"=w5580:i16, "Parameter Cluster (Scaled)"=w5578:T76)  [unwired: 2 in, 2 out]
        n3418 = local write "ET3500 Error"(w5579) -> ()
        n3419 = local write "Parameter Cluster (Scaled)"(w5578) -> ()
        n3420 = Merge Errors(w5579, w5577) -> (w5570:errorcluster)
        n3421 = control-ref of="WPS Details Setup"() -> (w5572:refnum<vi>)
        n3422 = control-ref of="Sequence Status"() -> (w5581:refnum<vi>)
        n3423 = control-ref of="MCListBox FHS Setup"() -> (w5582:refnum<vi>)
        n3424 = Unbundle By Name(w5578) -> ("PVIn (degC)"=w5583:dbl)
        n3425 = local read "TransactionRunNo"() -> (w5575:string)
        n3426 = local read "Transaction No"() -> (w5576:string)
        n3427 = property on="Current Temp" class="DigNum (strict)"("Value"=w5583) -> ()  [unwired: 2 in, 2 out]
        n3428 = local read "DB - Active Process"() -> (w5566:bool)
        n3429 = local read "DB - Transaction"() -> (w5574:bool)
        n3430 = flat-sequence {
          tunnel: w5570 -> [w5628]
          tunnel: [w5627] -> w5569
          tunnel: w5568 -> [w5644]
          tunnel: [w5641] -> w5565
          frame #0 {
            n3431 = while {
              tunnel: w5628 -> [w5639]
              tunnel: [w5638] -> w5627
              i -> [w5634]
              stop <- w5631 stop-if-true
              # "Check DAQ Started Flag"
              n3432 = local read "Simulate cRIO"() -> (w5637:bool)
              n3433 = local read "cRIO shared variable RT Library"() -> (w5629:string)
              n3434 = Wait Until Next ms Multiple(millisecond multiple=u32 100) -> ()  [unwired: 1 out]
              n3435 = Greater Or Equal?(x=w5634, y=50) -> (x >= y?=w5632:bool)
              n3436 = control-ref of="cRIO Status"() -> (w5635:refnum<vi>)
              n3437 = call "cRIO - Shared Variable RW.vi"("shared variable RT Library"=w5629, "Read/Write"=cRIO_RW_Enum."Read", "Error In"=w5639, "Simulate cRIO"=w5637, "cRIO Status"=w5635) -> ("DAQ Started"=w5630:bool, "Error Out"=w5638:errorcluster)  [unwired: 6 in, 7 out]
              n3438 = local write "cRIO DAQ Started"(w5630) -> ()
              n3439 = Or(x=w5630, y=w5632) -> (x .or. y?=w5631:bool)
              "Check DAQ Started Loop Count" <- w5634
            }
          }
          frame #1 {
            n3440 = local read "RecoveryFlag"() -> (w5645:bool)
            n3441 = And(x=w5644, y=w5645) -> (x .and. y?=w5643:bool)
            n3442 = case shown="True" w5643 {
              tunnel: [w5647 w5649] -> w5642
              tunnel: [w5646 w5648] -> w5641
              frame False {
                w5646 = 0  # Sample/ch Count = 0
                n3443 = Get Date/Time In Seconds() -> (seconds since 1Jan1904=w5647:timestamp)
              }
              frame True {
                # "20141010_115100.dat"
                # "c:\\temp\\SRTRS4070_Host\\Data_Host\\2014\\10\\106_20141010_115100.dat"
                # "cRIO DAQ already Started\nRecovery Mode"
                n3444 = local read "Raw Data File"() -> (w5654:string)
                n3445 = local read "Simulate cRIO"() -> (w5650:bool)
                n3446 = String To Path(string=w5654) -> (path=w5655:path)
                n3447 = case shown="True" w5650 {
                  tunnel: [w5657 w5658] -> w5648
                  frame False {
                    w5657 = 0  # Sample/ch Count = 0
                  }
                  frame True {
                    # "Each Sample is 60 sec or 1 count"
                    # "Continue TimeStamp from Last count"
                    n3448 = local read "Recovered Data Size"() -> (w5660:i32[])
                    n3449 = Index Array(array=w5660) -> (element=w5659:i32)  [unwired: 1 in]
                    n3450 = Increment(x=w5659) -> (x+1=w5658:i32)
                  }
                }
                n3451 = Strip Path(path=w5655) -> (name=w5653:string)  [unwired: 1 out]
                n3452 = Match Pattern(string=w5653, regular expression="_") -> (after substring=w5651:string)  [unwired: 1 in, 3 out]
                n3453 = call "String - Convert Str (YYYYmmdd_HHMMSS) to TimeStamp.vi"("YYYYmmdd_HHMMSS"=w5651) -> ("time stamp"=w5649:timestamp)  [unwired: 8 in, 2 out]
                n3454 = local write "RecoveryFlag"(FALSE ("RecoveryFlag")) -> ()
              }
            }
            "Process t0" <- w5642
          }
        }
        n3455 = Bundle("Transaction No"=w5576, "TransactionRunNo"=w5575) -> (w5573:T61)  [unwired: 1 in]
        n3456 = call "Status - Update Sequence Status.vi"("Sequence Status"=w5581, "WPS Details"=w5572, "DB - Transaction"=w5574, "Transaction"=w5573, "MCListBox FHS Setup"=w5582, "ET3504 Status"=w5567, "Error In"=w5579, "Parameter Cluster (Scaled)"=w5578, "DB - Active Process"=w5566, "Segment.Type"=w5580) -> ("Error Out"=w5571:errorcluster)  [unwired: 4 in, 1 out]
        n3457 = local write "cRIO Error"(w5569) -> ()
        n3458 = local write "System Status"(w5571) -> ()
      }
      frame "RUNNING Process" {
        # "Start at 1st call\nNo need to wait\nfor Timer"
        # "Should be 60s"
        n3459 = local read "Simulate cRIO"() -> (w5663:bool)
        n3460 = case shown="True" w5663 {
          tunnel: [w5686 w5690] -> w5662
          tunnel: w5661 -> [_ w5687]
          frame False {
            n3461 = Get Date/Time In Seconds() -> (seconds since 1Jan1904=w5686:timestamp)
          }
          frame True {
            # "Every count is 60sec"
            n3462 = local read "Process t0"() -> (w5691:timestamp)
            n3463 = Multiply(x=w5687, y=60) -> (x*y=w5688:i32)
            n3464 = Add(x=w5688, y=w5691) -> (x+y=w5690:timestamp)
          }
        }
        "Simulated TimeStamp" <- w5662
        n3465 = local read "Host Sampling Interval (s)"() -> (w5668:dbl)
        n3466 = local read "Process t0"() -> (w5681:timestamp)
        n3467 = Equal To 0?(x=w5661) -> (x = 0?=w5674:bool)
        n3468 = call "Elapsed Time"("Time Target (s)"=w5668) -> ("Elapsed Time (s)"=w5680:dbl, "Time has Elapsed"=w5677:bool)  [unwired: 11 in, 6 out]
        "Time has Elapsed" <- w5677
        n3469 = Subtract(x=w5662, y=w5681) -> (x-y=w5664:dbl)
        n3470 = Or(x=w5677, y=w5674) -> (x .or. y?=w5666:bool)
        n3471 = Subtract(x=w5668, y=w5680) -> (x-y=w5679:dbl)
        n3472 = Max & Min(x=0.0, y=w5679) -> (max(x,y)=→"Time to next sample (s)":dbl)  [unwired: 1 out]
        n3473 = case shown="True" w5666 {
          tunnel: w5664 -> [_ w6097]
          tunnel: [_ w6082] -> w5671
          tunnel: w5661 -> [w6041 w6072]
          tunnel: [w6041 w6078] -> w5678
          tunnel: [_ w6057] -> w5669
          frame False {
            # "Not Time Yet => SKIP Logging Of Data"
          }
          frame True {
            w6077 = 0.0  # Log Entry Offset
            w6102 = "," ("delimiter (Tab)")
            # "Add \\r\\n if no data from cRIO"
            # "#     hide zeroes\n_4   4 significant digits"
            # "in Minutes"
            # "New Data\nDelimiter is ,"
            n3474 = local read "Display Reference Chart"() -> (w6045:bool)
            n3475 = disable-structure shown="Disabled" {
              frame Disabled {
                n3476 = local read "Raw Data File"() -> ()  [unwired: 1 out]
              }
              frame Enabled {
              }
            }
            n3477 = local read "DB - Active Process"() -> (w6064:bool)
            n3478 = local read "Enable Central Monitoring"() -> (w6066:bool)
            n3479 = And(x=w6066, y=w6064) -> (x .and. y?=w6065:bool)
            n3480 = control-ref of="cRIO Status"() -> (w6058:refnum<vi>)
            n3481 = local read "Simulate cRIO"() -> (w6070:bool)
            n3482 = local read "cRIO shared variable RT Library"() -> (w6093:string)
            n3483 = global read "Global SRTRS.vi" "Logon"() -> (w6053:T21)
            n3484 = local read "cRIO Error"() -> (w6094:errorcluster)
            n3485 = Unbundle By Name(w6053) -> ("PlantID"=w6054:string, "SystemID"=w6055:string)
            n3486 = call "cRIO - Shared Variable RW.vi"("shared variable RT Library"=w6093, "Read/Write"=cRIO_RW_Enum."Read", "Error In"=w6094, "Simulate cRIO"=w6070, "cRIO Status"=w6058) -> ("File IO Status"=w6075:bool[], "Probe List Out"=w6096:i32[], "data out"=w6079:dbl[], "cRIO Timestamp"=w6090:timestamp, "Cycle Count"=w6098:i32, "DAQ Started"=w6095:bool, "Error Out"=w6087:errorcluster)  [unwired: 6 in, 2 out]
            "cRIO File IO Status (updated at File creation only)" <- w6075
            n3487 = Number To Decimal String(number=w6096) -> (decimal integer string=w6047:string[])  [unwired: 1 in]
            n3488 = case shown="True" w6045 {
              tunnel: w6047 -> [w6104 w6107]
              tunnel: [w6104 w6106] -> w6046
              frame False {
              }
              frame True {
                n3489 = Build Array (concatenate)(w6107, "Ref.") -> (w6106:string[])
              }
            }
            n3490 = for {
              tunnel: w6046 -> [w6191] mode=indexing
              i -> [w6192]
              n3491 = property on="Chart" class="WFChart (strict)"("Active Plot"=w6192, "Plot.Plot Name"=w6191) -> ()  [unwired: 2 in, 2 out]
            }
            n3492 = Bundle("PlantID"=w6054, "SystemID"=w6055) -> (w6052:cluster{"PlantID":string, "SystemID":string})  [unwired: 1 in]
            n3493 = local write "cRIO Timestamp"(w6090) -> ()
            n3494 = local write "cRIO Cycle Count"(w6098) -> ()
            n3495 = local write "cRIO DAQ Started"(w6095) -> ()
            n3496 = local read "Display Reference Chart"() -> (w6048:bool)
            n3497 = Select(t=errorcluster {"status"=TRUE, "code"=-1000, "source"="Simulate cRIO Comm Error. "} ("Error Out"), s="Simulate cRIO Comm Error", f=w6087) -> (s? t:f=w6057:errorcluster)
            n3498 = Select(t=dbl[] [], s="Simulate cRIO No Data", f=w6079) -> (s? t:f=w6044:dbl[])
            n3499 = Add(x=w6077, y=w6097) -> (x+y=w6092:dbl)
            n3500 = call "Status - Update cRIO Status.vi"("Error In"=w6057, "[PlantId],[SystemId]"=w6052, "cRIO Status"=w6058) -> ("Error Out"=w6056:errorcluster)  [unwired: 8 in]
            n3501 = local write "System Status"(w6056) -> ()
            n3502 = Divide(x=w6092, y=60.0) -> (x/y=w6050:dbl)
            n3503 = Index Array(array=w6044) -> (element=→"1st TC":dbl)  [unwired: 1 in]
            n3504 = local write "cRIO Error"(w6057) -> ()
            n3505 = local read "Simulate cRIO"() -> (w6069:bool)
            n3506 = Equal To 0?(x=w6072) -> (x = 0?=w6073:bool)
            n3507 = local read "DB - Transaction"() -> (w6074:bool)
            n3508 = And(x=w6074, y=w6073) -> (x .and. y?=w6071:bool)
            n3509 = Array Size(array=w6044) -> (size(s)=w6086:i32)
            n3510 = case shown="True" w6071 {
              tunnel: w6044 -> [_ w6156]
              frame False {
              }
              frame True {
                w6155 = T62[] [enum."[StartRecordTemp]", enum."[UnitOfTemperature]"] items=["[StartRecordTime]", "[StartRecordTemp]", "[MaxRecordedTemp]", "[MaxRecordedTempTime]", "[MinRecordedTemp]", "[MinRecordedTempTime]", "[EndRecordTemp]", "[EndRecordTime]", "[RecordedMinutes]", "[StartHoldTime]", "[StartHoldTemp]", "[HoldTimeMaxTemp]", "[HoldTimeMaxTempTime]", "[HoldTimeMinTemp]", "[HoldTimeMinTempTime]", "[EndHoldTime]", "[EndHoldTemp]", "[HoldDurationMinutes]", "[TempDiffDuringHold]", "[UnitOfTemperature]", "[PerformedBy]", "[PerformedOn]", "[IsTempWithinTol]", "[IsTimeWithinTol]", "[HoldTimePercentage]", "[ProcessStatus]", "[OverallStatus]", "[SequenceStatus]", "[Parameter1]", "[Parameter2]", "[Parameter3]", "[Parameter4]", "[Parameter5]", "[Parameter6]", "[Parameter7]", "[Parameter8]", "[Parameter9]", "[Parameter10]", "[Parameter11]", "[Parameter12]", "[Result]", "[RawDataFile]", "[RawDataFilePath]", "[RawDataFileName]", "[OutputSetId]", "[SavedBy]", "[SavedOn]", "[Inactive]"]  # [TransactionResult] v02
                # "Start Recording Temperature @ Sample/ch count = 0"
                n3511 = Index Array(array=w6156) -> (element=w6152:dbl)  [unwired: 1 in]
                n3512 = disable-structure shown="Enabled" {
                  frame Disabled {
                    n3513 = property on="Chart" class="WFChart (strict)"("XScale.Maximum"=600.0) -> ()  [unwired: 2 in, 2 out]
                  }
                  frame Enabled {
                  }
                }
                n3514 = property on="Info. Temperature Units" class="Str"() -> ("Value"=w6141:string)  [unwired: 2 in, 2 out]
                n3515 = Format Value(format string="%#_4", value (0)=w6152) -> (output string=w6151:string)  [unwired: 1 in]
                n3516 = Build Array(w6151, w6141) -> (w6144:string[])
                n3517 = local read "TransactionRunNo"() -> (w6149:string)
                n3518 = local read "Transaction No"() -> (w6150:string)
                n3519 = Bundle("Transaction No"=w6150, "TransactionRunNo"=w6149) -> (w6148:T61)  [unwired: 1 in]
                n3520 = call "DB - [Execute].[Transaction].vi"("DB.Schema.Table"="SRTRS.Execute.TransactionResult", "Transaction"=w6148, "DB - Execute Transaction"=DB_-_Execute_Transaction_Enum."UPDATE [TransactionResult]" ("DB - Setup Item Enum"), "[TransactionResult] v02"=w6155, "<Values>"=w6144) -> ("SUMMARY"=w6143:errorcluster)  [unwired: 11 in, 3 out]
                n3521 = local read "Enable Central Monitoring"() -> (w6146:bool)
                n3522 = local read "DB - Active Process"() -> (w6147:bool)
                n3523 = Build Array(w6141) -> (w6142:string[])
                n3524 = And(x=w6147, y=w6146) -> (x .and. y?=w6145:bool)
                n3525 = case shown="True" w6145 {
                  tunnel: w6142 -> [_ w6163]
                  tunnel: w6143 -> [_ w6162]
                  frame False {
                  }
                  frame True {
                    w6168 = T63[] [enum."[UnitOfTemperature]"] items=["[IsActive]", "[TransactionNo]", "[TransactionRunNo]", "[SequenceStatus]", "[StartRecordTime]", "[EndRecordTime]", "[StartHoldTime]", "[EndHoldTime]", "[Message1]", "[Message2]", "[HoldTimeRemaining]", "[HoldTimePercentage]", "[HoldProgressColor]", "[OrderNumbers]", "[CurrentTemp]", "[UnitOfTemperature]", "[IsAppClientLive]", "[RawDataFile]", "[RecordedMinutes]", "[FurnaceControlStatus]", "[FurnaceControlColor]", "[ControllerStatus]", "[ControllerColor]", "[IsControllerOnline]", "[ProcessColor]", "[OverallColor]", "[LastUpdatedOn]", "[LastUpdatedCmsTime]", "[Inactive]"] ("[Execute].[ActiveProcess]\n2014-10-14 14:58")
                    n3526 = global read "Global SRTRS.vi" "Logon"() -> (w6164:T21)
                    n3527 = Unbundle By Name(w6164) -> ("PlantID"=w6165:string, "SystemID"=w6166:string)
                    n3528 = Bundle("PlantID"=w6165, "SystemID"=w6166) -> (w6160:cluster{"PlantID":string, "SystemID":string})  [unwired: 1 in]
                    n3529 = call "DB - [CMS].[Execute].[ActiveProcess].vi"("Application"="SRTRS", "[PlantId],[SystemId]"=w6160, "error in (no error)"=w6162, "DB - CMS Execute ActiveProcess"=T74."UPDATE [Execute].[ActiveProcess]" ("DB - Execute ActiveProcess"), "[Execute].[ActiveProcess]\n2014-10-14 14:58"=w6168, "<Data>"=w6163) -> ("SUMMARY"=w6161:errorcluster)  [unwired: 10 in, 3 out]
                    n3530 = local write "DB"(w6161) -> ()
                  }
                }
              }
            }
            n3531 = Number To Fractional String(number=w6050, precision (6)=i16 1) -> (F-format string=w6101:string)  [unwired: 2 in]
            n3532 = Array To Spreadsheet String(delimiter (Tab)=w6102, array=w6044, 3:"%#_4" ("format string")) -> (spreadsheet string=w6103:string)
            n3533 = Greater Than 0?(x=w6086) -> (x > 0?=w6042:bool)
            n3534 = And(x=w6048, y=w6042) -> (x .and. y?=w6043:bool)
            n3535 = case shown="True" w6043 {
              tunnel: w6050 -> [_ w6112]
              tunnel: w6044 -> [w6108 w6111]
              tunnel: [w6108 w6109] -> w6049
              frame False {
              }
              frame True {
                n3536 = call "ET3500 - Reference Profile Pt-by-Pt.vi"("Time (sec)"=w6112) -> ("Ref Temperature"=w6110:dbl)  [unwired: 3 in, 1 out]
                n3537 = Build Array (concatenate)(w6111, w6110) -> (w6109:dbl[])
              }
            }
            n3538 = call "Convert to Dynamic Data"("Array"=w6049) -> ("Dynamic Data Type"=w6068:dynamicdata)  [unwired: 3 in]
            n3539 = case shown="False" w6069 {
              tunnel: w6068 -> [w6119 w6123]
              tunnel: [w6119 w6120] -> w6067
              frame False {
              }
              frame True {
                n3540 = local read "Simulated TimeStamp"() -> (w6121:timestamp)
                n3541 = for {
                  N: 8 -> [_]
                  shift-right: [w6126] -> w6120
                  shift-left: w6123 -> [w6127]
                  tunnel: w6121 -> [w6124]
                  i -> [w6125]
                  n3542 = xnode ("Set Dynamic Data Attributes")("Signals In"=w6127, "Signal Index"=w6125, "Timestamp"=w6124) -> ("Signals Out"=w6126:dynamicdata)  [unwired: 1 in, 1 out]
                }
              }
            }
            "Chart" <- w6067
            n3543 = Concatenate Strings(w6101, w6102, w6103) -> (w6083:string)
            n3544 = Concatenate Strings(w6083, "\r\n" ("string")) -> (w6085:string)
            n3545 = local read "Logged File Ref"() -> (w6062:refnum<file>)
            n3546 = Select(t=w6083, s=w6042, f=w6085) -> (s? t:f=w6051:string)
            n3547 = case shown="True" w6065 {
              tunnel: w6052 -> [_ w6117]
              tunnel: w6051 -> [_ w6116]
              frame False {
              }
              frame True {
                w6115 = "NULL"  # End of FileStream (NULL)
                n3548 = call "DB - [CMS].[Execute].[ActiveProcess].vi"("Application"="SRTRS", "String ([RawDataFile] Filestream)"=w6116, "[PlantId],[SystemId]"=w6117, "Filestream Position (0/<int>/NULL)"=w6115, "DB - CMS Execute ActiveProcess"=DB_-_CMS_Execute_Active_Process."UPDATE FILESTREAM") -> ("SUMMARY"=w6118:errorcluster)  [unwired: 11 in, 3 out]
                n3549 = local write "DB"(w6118) -> ()
              }
            }
            n3550 = Set File Position(refnum=w6062, from (0:start)=enum16{"start", "end", "current"}."end") -> (refnum out=w6061:refnum<file>, error out=w6059:errorcluster)  [unwired: 2 in]
            n3551 = Write to Text File(file (use dialog)=w6061, text=w6051, error in=w6059) -> (error out=w6082:errorcluster)  [unwired: 1 in, 2 out]
            n3552 = local write "Data File Error"(w6082) -> ()
            n3553 = case shown="True" w6042 {
              tunnel: w6072 -> [w6175 w6177]
              tunnel: [w6175 w6178] -> w6078
              tunnel: w6075 -> [_ w6176]
              frame False {
                # "Array = 0, cRIO No data"
                n3554 = Number To Decimal String(number=w6175) -> (decimal integer string=w6173:string)  [unwired: 1 in]
                n3555 = Concatenate Strings("{Running Process} " ("element"), "cRIO No Data. Current Samples/ch Count = " ("element"), w6173, ". " ("string")) -> (w6170:string)
                n3556 = call "Queue - EnQueue to MessageQ.vi"("<NoD> Don't Display to UI"=TRUE, "Message"=w6170) -> ()  [unwired: 9 in, 1 out]
              }
              frame True {
                # "Samples/ch Count +1"
                # "Array >0 , cRIO Data OK"
